vi "GetControlReference.vi"(1 "element":string="output cluster", 2 "Controls[]":refnum<vi>[](array[refnum])) -> (0 "Control Out":refnum<vi>)   [LabVIEW 2018]
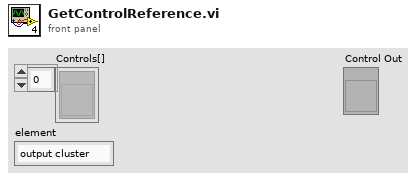
[diagram p1: front panel]
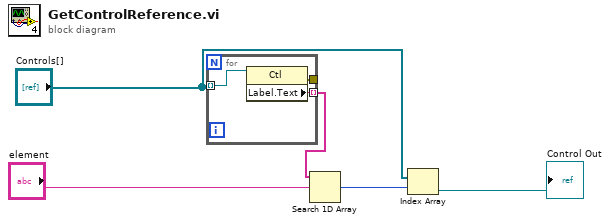
[diagram p0: block diagram]
diagram:
  n1 = for {
    tunnel: "Controls[]" -> [w6] mode=indexing
    tunnel: [w8] -> w3 mode=indexing
    tunnel: [w7] -> _
    n2 = property class="Ctl"(reference=w6) -> (error out=w7:errorcluster, "Label.Text"=w8:string)  [unwired: 1 in, 1 out]
  }
  n3 = Search 1D Array(1D array=w3, element="element") -> (index of element=w5:i32)  [unwired: 1 in]
  n4 = Index Array(array="Controls[]", index=w5) -> (element=→"Control Out":refnum<vi>)
